vi "SimpleExamples.vi"() -> ()   [LabVIEW 2013]
panel:
  out "Returned Cluster Wrapping Array":T1
  out "Some Cluster Returned 2":T2
  in  "Some Cluster 2":T2={"A"=200, "B"=123, "C"=789, {"E"=0.222, "F"=9999}, "G"=4.567, "H"=89}
  in  "Some Cluster":T2={"A"=200, "B"=123, "C"=789, {"E"=0.222, "F"=9999}, "G"=4.567, "H"=89}
  out "Some Cluster Returned":T2
  out "Array from Memory Location":cluster{"X":dbl, "Y":dbl}[](array[cluster])
  # "### BSD License (http://www.opensource.org/licenses/bsd-license.php) Begin ###\n \nCopyright (c) 2014 Jeffrey Holt <jolt.holt@gmail.com>\n\nAll rights reserved.\n\nRedistribution and use in source and binary forms, with or without modification, are permitted provided that the following conditions are met:\n\n    * Redistributions of source code must retain the above copyright notice\n\nTHIS SOFTWARE IS PROVIDED BY THE COPYRIGHT HOLDERS AND CONTRIBUTORS \"AS IS\" AND ANY EXPRESS OR IMPLIED WARRANTIES, \nINCLUDING, BUT NOT LIMITED TO, THE IMPLIED WARRANTIES OF MERCHANTABILITY AND FITNESS FOR A PARTICULAR PURPOSE ARE \nDISCLAIMED. IN NO EVENT SHALL THE COPYRIGHT OWNER OR CONTRIBUTORS BE LIABLE FOR ANY DIRECT, INDIRECT, INCIDENTAL,\n SPECIAL, EXEMPLARY, OR CONSEQUENTIAL DAMAGES (INCLUDING, BUT NOT LIMITED TO, PROCUREMENT OF SUBSTITUTE GOODS OR \nSERVICES; LOSS OF USE, DATA, OR PROFITS; OR BUSINESS INTERRUPTION) HOWEVER CAUSED AND ON ANY THEORY OF LIABILITY, \nWHETHER IN CONTRACT, STRICT LIABILITY, OR TORT (INCLUDING NEGLIGENCE OR OTHERWISE) ARISING IN ANY WAY OUT OF THE USE \nOF THIS SOFTWARE, EVEN IF ADVISED OF THE POSSIBILITY OF SUCH DAMAGE.\n\n### BSD License End ###"
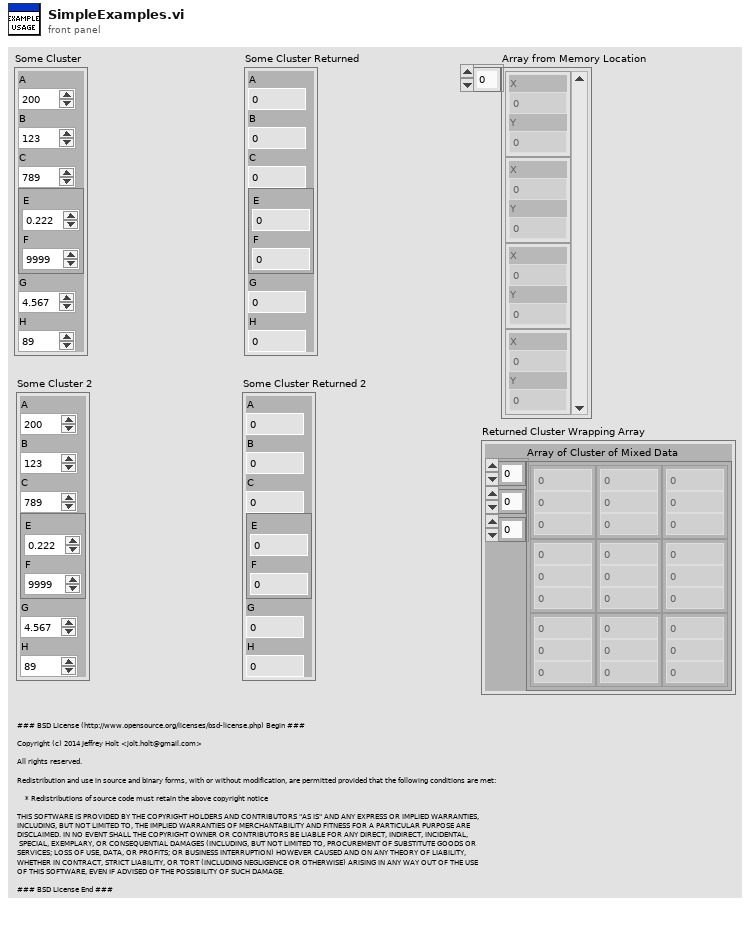
[diagram p1: front panel]
types:
  T1 = cluster{"Array of Cluster of Mixed Data":cluster{i32, dbl, i32}[][][]}
  T2 = cluster{"A":u8, "B":i32, "C":i32, cluster{"E":dbl, "F":i32}, "G":dbl, "H":i32}
  T3 = cluster{"Multi Dimension Mixed Data Array":cluster{i32, dbl, i32}[][][]}
  T4 = enum16{"big-endian, network order", "native, host order", "little-endian"}
  T5 = typedef "ctl_ElementAndPaddingInfo.ctl" = cluster{"Data Mask":bool[], "Data Element Info":T6[]}
  T6 = typedef "ctl_DataElementInfo.ctl" = cluster{"Type":u16, "Num Bytes Removed":u16, "Org Size (flattened string)":i32, "Removed Bytes":u8[]}
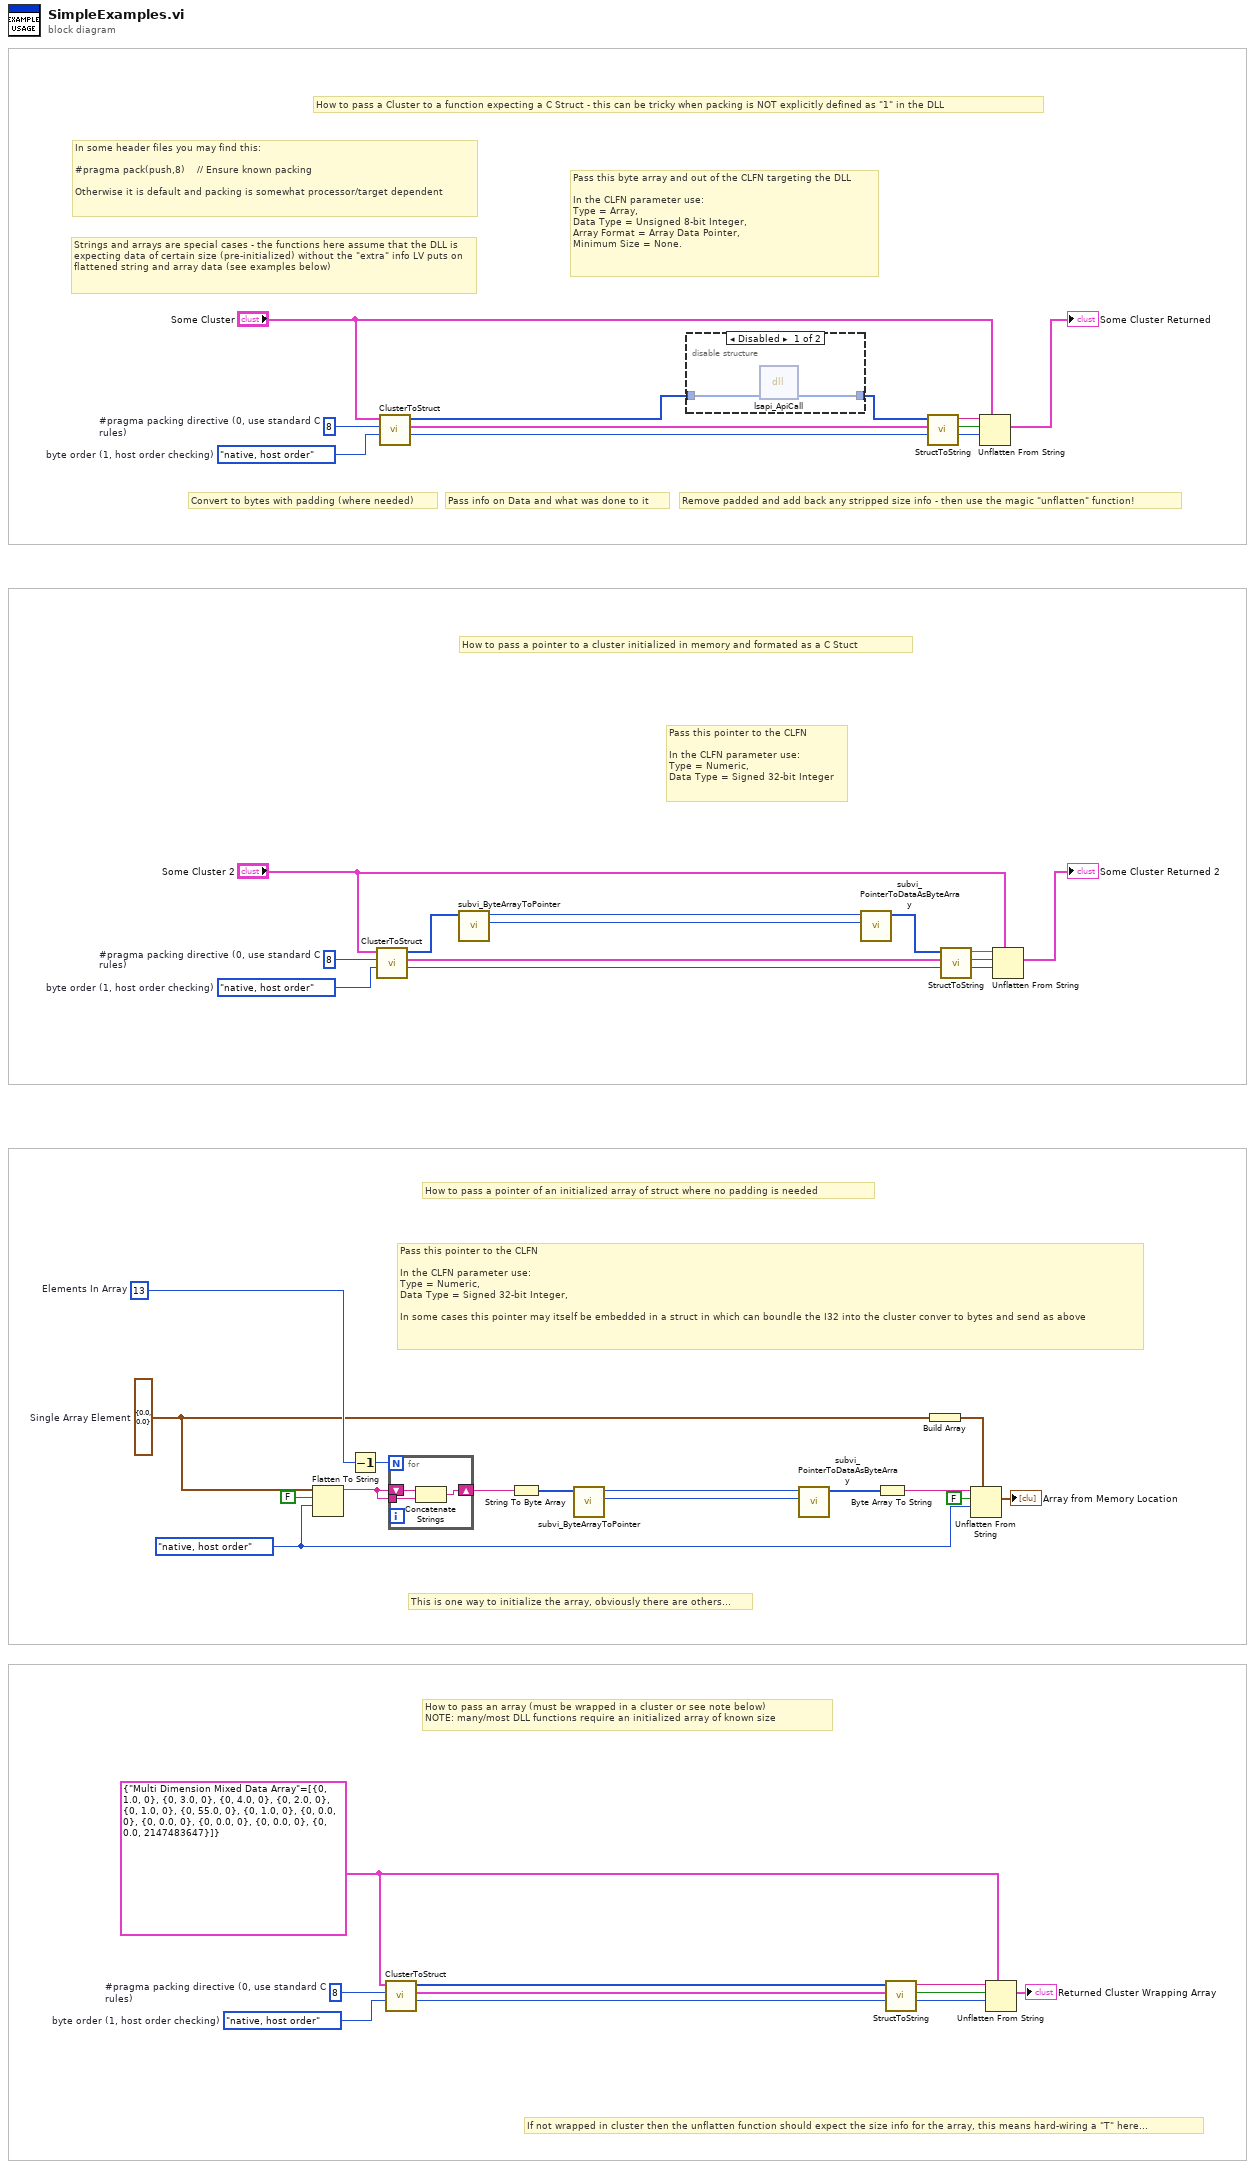
[diagram p0: block diagram]
diagram:
  w5 = T3 {"Multi Dimension Mixed Data Array"=[[[{0, 1.0, 0}, {0, 3.0, 0}, {0, 4.0, 0}], [{0, 2.0, 0}, {0, 1.0, 0}, {0, 55.0, 0}]], [[{0, 1.0, 0}, {0, 0.0, 0}, {0, 0.0, 0}], [{0, 0.0, 0}, {0, 0.0, 0}, {0, 0.0, 2147483647}]]]}
  w12 = T4."native, host order"  # byte order (1, host order checking)
  w11 = 8  # #pragma packing directive (0, use standard C rules)
  w14 = T4."native, host order"  # byte order (1, host order checking)
  w15 = 8  # #pragma packing directive (0, use standard C rules)
  w27 = T4."native, host order"  # byte order (1, host order checking)
  w28 = 8  # #pragma packing directive (0, use standard C rules)
  w41 = T4."native, host order" ("byte order (0:big-endian, network order)")
  w39 = 13  # Elements In Array
  w38 = cluster{"X":dbl, "Y":dbl} {"X"=0.0, "Y"=0.0}  # Single Array Element
  # "Strings and arrays are special cases - the functions here assume that the DLL is expecting data of certain size (pre-initialized) without the \"extra\" info LV puts on flattened string and array data (see examples below)"
  # "Remove padded and add back any stripped size info - then use the magic \"unflatten\" function!"
  # "Pass info on Data and what was done to it"
  # "Convert to bytes with padding (where needed)"
  # "If not wrapped in cluster then the unflatten function should expect the size info for the array, this means hard-wiring a \"T\" here..."
  # "How to pass an array (must be wrapped in a cluster or see note below)\nNOTE: many/most DLL functions require an initialized array of known size"
  # "This is one way to initialize the array, obviously there are others..."
  # "Pass this pointer to the CLFN\n\nIn the CLFN parameter use:\nType = Numeric,\nData Type = Signed 32-bit Integer"
  # "How to pass a pointer to a cluster initialized in memory and formated as a C Stuct"
  # "How to pass a Cluster to a function expecting a C Struct - this can be tricky when packing is NOT explicitly defined as \"1\" in the DLL"
  # "Pass this pointer to the CLFN\n\nIn the CLFN parameter use:\nType = Numeric,\nData Type = Signed 32-bit Integer,\n\nIn some cases this pointer may itself be embedded in a struct in which can boundle the I32 into the cluster conver to bytes and send as above"
  # "In some header files you may find this:\n\n#pragma pack(push,8)    // Ensure known packing\n\nOtherwise it is default and packing is somewhat processor/target dependent"
  # "Pass this byte array and out of the CLFN targeting the DLL\n\nIn the CLFN parameter use:\nType = Array,\nData Type = Unsigned 8-bit Integer,\nArray Format = Array Data Pointer,\nMinimum Size = None."
  # "How to pass a pointer of an initialized array of struct where no padding is needed"
  n1 = Flatten To String(anything=w38, prepend array or string size? (T)=FALSE, byte order (0:big-endian, network order)=w41) -> (data string=w49:string)  [unwired: 1 in, 2 out]
  n2 = Decrement(x=w39) -> (x-1=w48:i32)
  n3 = call "ClusterToStruct.vi"("byte order (1, host order checking)"=w14, "#pragma packing directive (0, default)"=w15, "LV Cluster"="Some Cluster 2") -> ("byte order Used"=w23:T4, "Element and Padding Info"=w22:T5, "Cluster Data as Byte Array Out"=w24:u8[])  [unwired: 4 in, 2 out]
  n4 = call "ClusterToStruct.vi"("byte order (1, host order checking)"=w27, "#pragma packing directive (0, default)"=w28, "LV Cluster"="Some Cluster") -> ("byte order Used"=w34:T4, "Element and Padding Info"=w33:T5, "Cluster Data as Byte Array Out"=w2:u8[])  [unwired: 4 in, 2 out]
  n5 = call "ClusterToStruct.vi"("byte order (1, host order checking)"=w12, "#pragma packing directive (0, default)"=w11, "LV Cluster"=w5) -> ("byte order Used"=w6:T4, "Element and Padding Info"=w7:T5, "Cluster Data as Byte Array Out"=w10:u8[])  [unwired: 4 in, 2 out]
  n6 = for {
    N: w48 -> [_]
    shift-right: [w50] -> w47
    shift-left: w49 -> [w52]
    tunnel: w49 -> [w51]
    n7 = Concatenate Strings(w52, w51) -> (w50:string)
  }
  n8 = call "subvi_ByteArrayToPointer.vi"("Byte Array In"=w24) -> ("Size"=w25:i32, "Pointer"=w17:i32)  [unwired: 8 in, 1 out]
  n9 = String To Byte Array(string=w47) -> (unsigned byte array=w46:u8[])
  n10 = call "subvi_ByteArrayToPointer.vi"("Byte Array In"=w46) -> ("Size"=w35:i32, "Pointer"=w45:i32)  [unwired: 8 in, 1 out]
  n11 = disable-structure shown="Disabled" {
    disable-tunnel: w2 -> [w54 w55]
    disable-tunnel: [w53 w55] -> w1
    frame Disabled {
      n12 = dll-call lib="?" fn="lsapi_ApiCall" label="Call Library Function Node"("ApiCallHdr"=w54) -> ("ApiCallHdr"=w53:u8[])  [unwired: 4 in, 2 out]
    }
    frame Enabled {
    }
  }
  n13 = call "subvi_PointerToDataAsByteArray.vi"("Size"=w35, "Pointer"=w45) -> ("Byte Array Out"=w40:u8[])  [unwired: 8 in, 1 out]
  n14 = call "subvi_PointerToDataAsByteArray.vi"("Size"=w25, "Pointer"=w17) -> ("Byte Array Out"=w21:u8[])  [unwired: 8 in, 1 out]
  n15 = Byte Array To String(unsigned byte array=w40) -> (string=w44:string)
  n16 = call "StructToString.vi"("byte order"=w6, "Element and Padding Info"=w7, "Data as Unsigned Byte Array (with padding)"=w10) -> ("byte order (0:big-endian, network order) 2"=w9:T4, "Size Included (Always F)"=w3:bool, "Data As String for Unflatten Function"=w8:string)  [unwired: 5 in, 1 out]
  n17 = call "StructToString.vi"("byte order"=w34, "Element and Padding Info"=w33, "Data as Unsigned Byte Array (with padding)"=w1) -> ("byte order (0:big-endian, network order) 2"=w30:T4, "Size Included (Always F)"=w32:bool, "Data As String for Unflatten Function"=w31:string)  [unwired: 5 in, 1 out]
  n18 = Build Array(w38) -> (w37:cluster{"X":dbl, "Y":dbl}[])
  n19 = call "StructToString.vi"("byte order"=w23, "Element and Padding Info"=w22, "Data as Unsigned Byte Array (with padding)"=w21) -> ("byte order (0:big-endian, network order) 2"=w18:T4, "Size Included (Always F)"=w20:bool, "Data As String for Unflatten Function"=w19:string)  [unwired: 5 in, 1 out]
  n20 = Unflatten From String(type=w37, binary string=w44, data includes array or string size? (T)=FALSE, byte order (0:big-endian, network order)=w41) -> (value=→"Array from Memory Location":cluster{"X":dbl, "Y":dbl}[])  [unwired: 1 in, 2 out]
  n21 = Unflatten From String(type="Some Cluster", binary string=w31, data includes array or string size? (T)=w32, byte order (0:big-endian, network order)=w30) -> (value=→"Some Cluster Returned":T2)  [unwired: 1 in, 2 out]
  n22 = Unflatten From String(type=w5, binary string=w8, data includes array or string size? (T)=w3, byte order (0:big-endian, network order)=w9) -> (value=→"Returned Cluster Wrapping Array":T3)  [unwired: 1 in, 2 out]
  n23 = Unflatten From String(type="Some Cluster 2", binary string=w19, data includes array or string size? (T)=w20, byte order (0:big-endian, network order)=w18) -> (value=→"Some Cluster Returned 2":T2)  [unwired: 1 in, 2 out]
